vi "ScanSafetyStatus.vi"(11 "safetyStatus in":string) -> (3 "safetyStatus out":T1)   [LabVIEW 2016, in "Universal Robot.lvclass"]
uses:
  Universal Robot.lvclass
  SafetyStatus.ctl
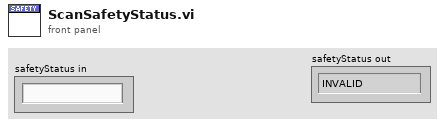
[diagram p1: front panel]
types:
  T1 = typedef "Universal Robot.lvclass/SafetyStatus.ctl" = enum16{"INVALID", "NORMAL", "REDUCED", "PROTECTIVE_STOP", "RECOVERY", "SAFEGUARD_STOP", "SYSTEM_EMERGENCY_STOP", "ROBOT_EMERGENCY_STOP", "VIOLATION", "FAULT", "AUTOMATIC_MODE_SAFEGAURD_STOP", "SYSTEM_THREE_POSITION_ENABLING_STOP"}
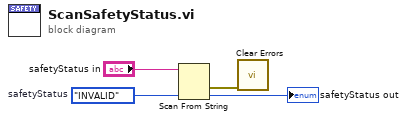
[diagram p0: block diagram]
diagram:
  w3 = SafetyStatus."INVALID"  # safetyStatus
  n1 = Scan From String(input string="safetyStatus in", default 1=w3) -> (error out=w1:errorcluster, output 1=→"safetyStatus out":T1)  [unwired: 3 in, 2 out]
  n2 = call <vilib>:"Clear Errors.vi"("error in (no error)"=w1) -> ()  [unwired: 5 in, 2 out]
